vi "LWConexCC_Close.vi"(3 "error in (no error)":errorcluster caption="error in", 5 "Conex CC Reference":refnum<k24>) -> (0 "Error out":errorcluster caption="error out")   [LabVIEW 2015]
uses:
  Newport.CONEXCC.CommandInterface
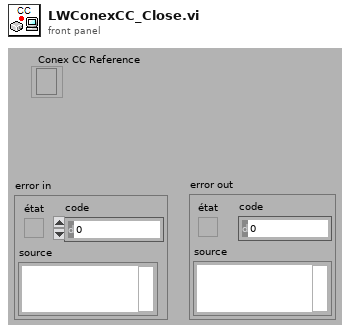
[diagram p1: front panel]
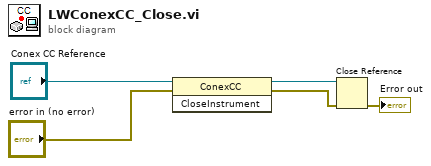
[diagram p0: block diagram]
diagram:
  n1 = invoke class="ConexCC" method="CloseInstrument"(reference="Conex CC Reference", error in="error in (no error)") -> (reference out=w5:refnum<k24>, error out=w4:errorcluster)  [unwired: 1 in, 1 out]
  n2 = Close Reference(reference=w5, error in (no error)=w4) -> (error out=→"Error out":errorcluster)
